vi "launchVI.vi"(8 "error in (no error)":errorcluster, 10 "UI.lvclass":refnum<class "UI.lvclass">, 11 "Panel in":refnum<class "Panel.lvclass">) -> (0 "error out":errorcluster, 2 "VI ref Out":refnum<vi>, 3 "Panel out":refnum<class "Panel.lvclass">)   [LabVIEW 2019, in "Panel.lvclass"]
uses:
  Panel.lvclass
  User Interface/UI.lvclass
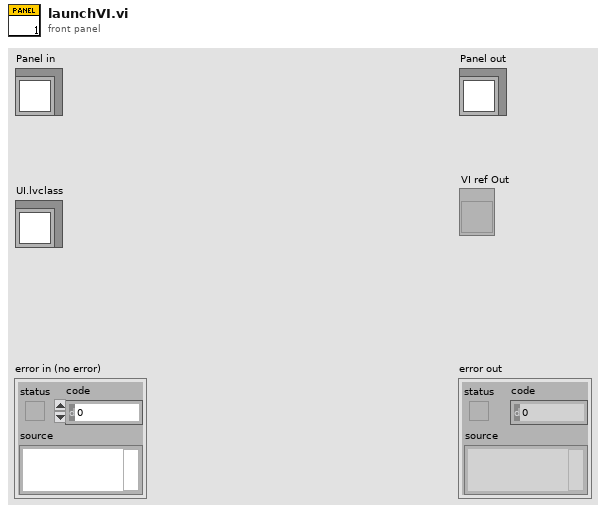
[diagram p1: front panel]
types:
  T1 = enum16{"Open Reference", "Launch VI", "Get VI Outputs"}
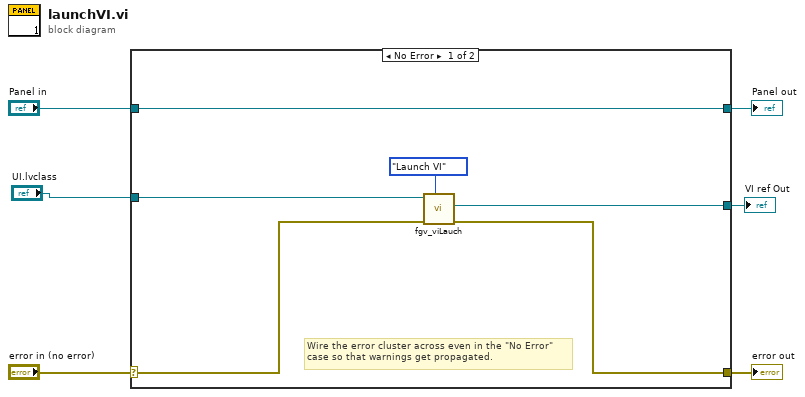
[diagram p0: block diagram]
diagram:
  n1 = case shown="No Error" "error in (no error)" {
    selector: "error in (no error)" -> [w9 w14]
    tunnel: [w8 w14] -> w5
    tunnel: [w12 w13] -> w3
    tunnel: "Panel in" -> [w12 w13]
    tunnel: "UI.lvclass" -> [w11 _]
    tunnel: [w7 _] -> w1
    frame No Error {
      # "Wire the error cluster across even in the \"No Error\"\ncase so that warnings get propagated."
      n2 = call "fgv_viLauch.vi"("Option"=T1."Launch VI", "Error In"=w9, "UI in"=w11) -> ("Error Out"=w8:errorcluster, "VI ref Out"=w7:refnum<vi>)  [unwired: 6 in, 1 out]
    }
    frame Error {
    }
  }
  "error out" <- w5
  "Panel out" <- w3
  "VI ref Out" <- w1
